vi "is_valid.vi"(8 "error in (no error)":errorcluster, 11 "DoublyNodeRef in":refnum<class "DoublyNodeRef.lvclass">) -> (0 "error out":errorcluster, 1 "valid?":bool, 3 "DoublyNodeRef out":refnum<class "DoublyNodeRef.lvclass">)   [LabVIEW 2021, in "DoublyNodeRef.lvclass"]
uses:
  DoublyNodeRef.lvclass
  DoublyNodeRef.lvclass/DoublyNodeRef.ctl
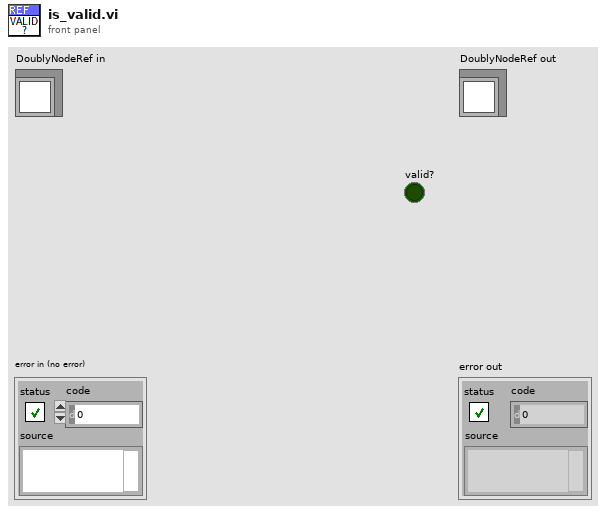
[diagram p1: front panel]
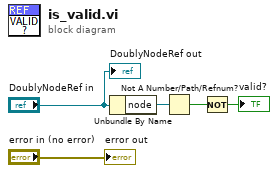
[diagram p0: block diagram]
diagram:
  n1 = Unbundle By Name("DoublyNodeRef in") -> ("node"=w3:refnum<data-value>)
  n2 = Not A Number/Path/Refnum?(number/path/refnum=w3) -> (NaN/Path/Refnum?=w2:bool)
  n3 = Not(x=w2) -> (.not. x?=→"valid?":bool)
  "error out" <- "error in (no error)"
  "DoublyNodeRef out" <- "DoublyNodeRef in"
